vi "Create.vi"(8 "error in (no error)":errorcluster, 11 "ref":refnum<k24>) -> (0 "error out":errorcluster, 3 "Query Result out":refnum<class "DapperResult.lvclass">)   [LabVIEW 2020, in "ORM_Dapper.lvlib" / "DapperResult.lvclass"]
uses:
  DapperResult.lvclass
  DapperResult.lvclass/DapperResult.ctl
  Write ref.vi
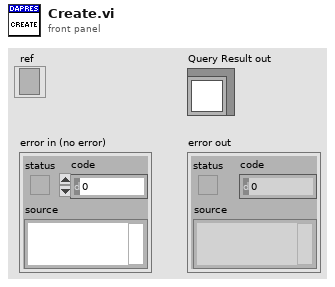
[diagram p1: front panel]
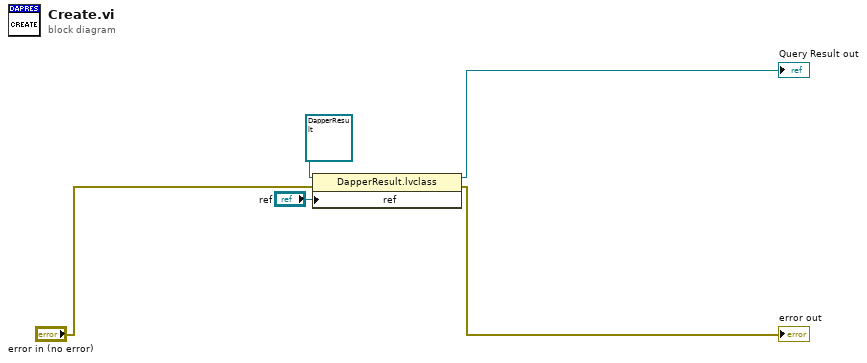
[diagram p0: block diagram]
diagram:
  n1 = property class="DapperResult.lvclass"(reference=refnum<class "DapperResult.lvclass"> refnum ("Query Result in"), error in="error in (no error)", "ref"="ref") -> (reference out=→"Query Result out":refnum<class "DapperResult.lvclass">, error out=→"error out":errorcluster)
